vi "runtest.vi"() -> ()   [LabVIEW 2016]
uses:
  <vilib>/addons/_JKI Toolkits/Caraya/run-tests/Run Test (Scalar Path).vi
  <vilib>/Wiresmith Technology/G CLI/CLI Class/CLI.lvclass
  <vilib>/addons/_JKI Toolkits/Caraya/Caraya.lvlib
panel:
  out "error out":errorcluster
  out "Application:Command Line Arguments":string[](array[string])
  out "recursive":bool
  out "verbose":bool
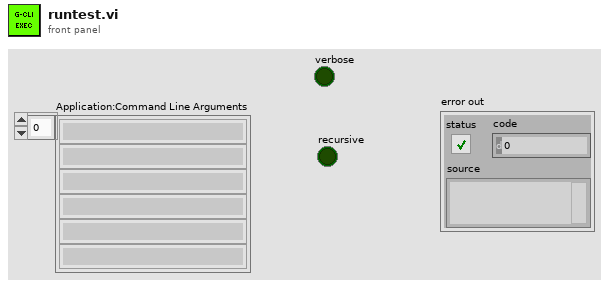
[diagram p1: front panel]
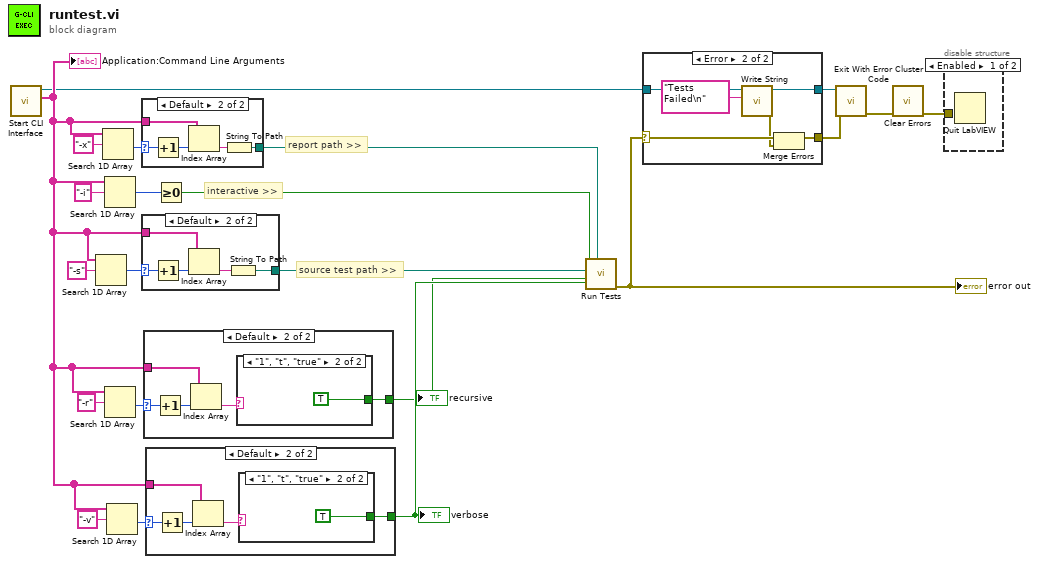
[diagram p0: block diagram]
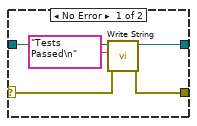
[diagram p3: hidden frame]
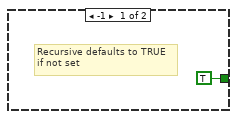
[diagram p6: hidden frame]
diagram:
  # "source test path >>"
  # "interactive >>"
  # "report path >>"
  n1 = call <vilib>:"Start CLI Interface.vi"() -> ("Custom Parameters"=w11:string[], "CLI out"=w10:refnum<class "CLI.lvclass">)  [unwired: 8 in, 2 out]
  "Application:Command Line Arguments" <- w11
  n2 = Search 1D Array(1D array=w11, element="-s") -> (index of element=w13:i32)  [unwired: 1 in]
  n3 = Search 1D Array(1D array=w11, element="-x") -> (index of element=w15:i32)  [unwired: 1 in]
  n4 = Search 1D Array(1D array=w11, element="-i") -> (index of element=w21:i32)  [unwired: 1 in]
  n5 = Search 1D Array(1D array=w11, element="-r") -> (index of element=w18:i32)  [unwired: 1 in]
  n6 = Search 1D Array(1D array=w11, element="-v") -> (index of element=w19:i32)  [unwired: 1 in]
  n7 = case shown="Default" w15 {
    selector: w15 -> [_ w26]
    tunnel: w11 -> [_ w25]
    tunnel: [_ w23] -> w8
    frame -1 {
    }
    frame Default {
      n8 = Increment(x=w26) -> (x+1=w27:i32)
      n9 = Index Array(array=w25, index=w27) -> (element=w24:string)
      n10 = String To Path(string=w24) -> (path=w23:path)
    }
  }
  n11 = case shown="Default" w13 {
    selector: w13 -> [_ w31]
    tunnel: w11 -> [_ w30]
    tunnel: [_ w28] -> w6
    frame -1 {
    }
    frame Default {
      n12 = Increment(x=w31) -> (x+1=w32:i32)
      n13 = Index Array(array=w30, index=w32) -> (element=w29:string)
      n14 = String To Path(string=w29) -> (path=w28:path)
    }
  }
  n15 = case shown="Default" w18 {
    selector: w18 -> [_ w35]
    tunnel: [TRUE w36] -> w5
    tunnel: w11 -> [_ w34]
    frame -1 {
      # "Recursive defaults to TRUE\nif not set"
    }
    frame Default {
      n16 = Increment(x=w35) -> (x+1=w38:i32)
      n17 = Index Array(array=w34, index=w38) -> (element=w37:string)
      n18 = case shown="\"1\", \"t\", \"true\"" w37 {
        tunnel: [_ TRUE] -> w36
        frame Default {
        }
        frame "1", "t", "true" {
        }
      }
    }
  }
  "recursive" <- w5
  n19 = case shown="Default" w19 {
    selector: w19 -> [_ w41]
    tunnel: [_ w42] -> w12
    tunnel: w11 -> [_ w40]
    frame -1 {
      # "Verosity defaults to False\nif not set"
    }
    frame Default {
      n20 = Increment(x=w41) -> (x+1=w44:i32)
      n21 = Index Array(array=w40, index=w44) -> (element=w43:string)
      n22 = case shown="\"1\", \"t\", \"true\"" w43 {
        tunnel: [_ TRUE] -> w42
        frame Default {
        }
        frame "1", "t", "true" {
        }
      }
    }
  }
  "verbose" <- w12
  n23 = Greater Or Equal To 0?(x=w21) -> (x >= 0?=w7:bool)
  n24 = call-poly <vilib>:"Run Tests.vi"("Verbose"=w12, "Report Path"=w8, "Inspect Recursively (T)"=w5, "Test Path"=w6, "Interactive (T)"=w7) -> ("error out"=w9:errorcluster)  [unwired: 5 in, 1 out]
  "error out" <- w9
  n25 = case shown="Error" w9 {
    selector: w9 -> [w47 w53]
    tunnel: w10 -> [w50 w56]
    tunnel: [w49 w55] -> w3
    tunnel: [w46 w51] -> w2
    frame No Error {
      n26 = call <vilib>:"Write String.vi"("error in (no error)"=w47, "Text to Write"="Tests Passed\n", "CLI in"=w50) -> ("error out"=w46:errorcluster, "CLI out"=w49:refnum<class "CLI.lvclass">)  [unwired: 7 in]
    }
    frame Error {
      n27 = call <vilib>:"Write String.vi"("Text to Write"="Tests Failed\n", "CLI in"=w56) -> ("error out"=w52:errorcluster, "CLI out"=w55:refnum<class "CLI.lvclass">)  [unwired: 8 in]
      n28 = Merge Errors(w53, w52) -> (w51:errorcluster)
    }
  }
  n29 = call <vilib>:"Exit With Error Cluster Code.vi"("error in (no error)"=w2, "CLI in"=w3) -> ("error out"=w4:errorcluster)  [unwired: 9 in]
  n30 = call <vilib>:"Clear Errors.vi"("error in (no error)"=w4) -> ("error out"=w1:errorcluster)  [unwired: 5 in, 1 out]
  n31 = disable-structure shown="Enabled" {
    disable-tunnel: w1 -> [_ _]
    frame Enabled {
      n32 = Quit LabVIEW() -> ()  [unwired: 1 in]
    }
    frame Disabled {
    }
  }
